vi "Launch Storage Line.vi"(8 "error in (no error)":errorcluster, 11 "cRIO-CO2 in":refnum<class "cRIO-CO2.lvclass">) -> (0 "error out":errorcluster, 3 "cRIO-CO2 out":refnum<class "cRIO-CO2.lvclass">)   [LabVIEW 2015, in "cRIO-Carbondioxide.lvlib" / "cRIO-CO2.lvlib" / "cRIO-CO2.lvclass"]
uses:
  cRIO-CO2.lvclass
  Storage Line/Storage Line.lvclass
  CO2 Actor/CO2 Actor.lvclass
  <vilib>/ActorFramework/Actor/Actor.lvclass
  cRIO-CO2.lvclass/cRIO-CO2.ctl
  cRIO-CO2 Messages/Log Message Msg/Log Message Msg.lvclass/Log Message Msg.ctl
  <vilib>/ActorFramework/Message Enqueuer/Message Enqueuer.lvclass/Message Enqueuer.ctl
  <vilib>/ActorFramework/Message Enqueuer/Enqueue.vi
  <vilib>/ActorFramework/Message Priority Queue/Priority Enqueue.vi
  <vilib>/ActorFramework/Message Enqueuer/Message Enqueuer.lvclass
  cRIO-CO2 Messages/Log Message Msg/Log Message Msg.lvclass
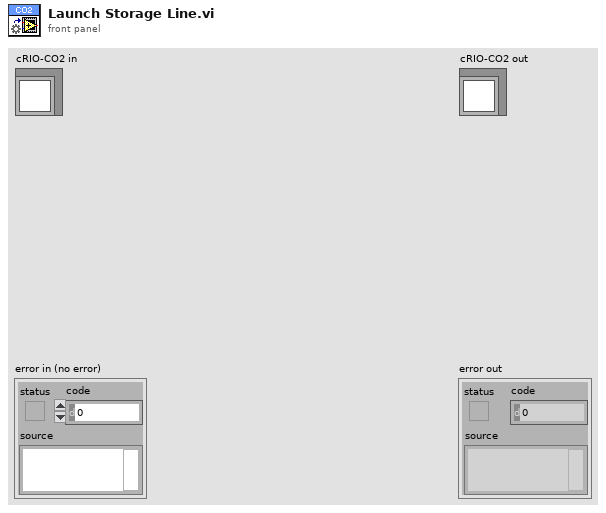
[diagram p1: front panel]
types:
  T1 = typedef "Dedicated Enqueuers.ctl" = cluster{"Freezers":cluster{"Syringe":refnum<class "Message Enqueuer.lvclass">, "Tank 1":refnum<class "Message Enqueuer.lvclass">, "Tank 2":refnum<class "Message Enqueuer.lvclass">, "Tank 3":refnum<class "Message Enqueuer.lvclass">, "Tank 4":refnum<class "Message Enqueuer.lvclass">}, "Heaters":cluster{"Syringe":refnum<class "Message Enqueuer.lvclass">, "Piston":refnum<class "Message Enqueuer.lvclass">}, "Blowers":cluster{"Tank 1":refnum<class "Message Enqueuer.lvclass">, "Tank 2":refnum<class "Message Enqueuer.lvclass">, "Tank 3":refnum<class "Message Enqueuer.lvclass">, "Tank 4":refnum<class "Message Enqueuer.lvclass">, "Syringe":refnum<class "Message Enqueuer.lvclass">}, "Sample Line":refnum<class "Message Enqueuer.lvclass">, "Storage Line":refnum<class "Message Enqueuer.lvclass">, "Transfer Line":refnum<class "Message Enqueuer.lvclass">, "Syringe Stepper":refnum<class "Message Enqueuer.lvclass">, "Syringe Line":refnum<class "Message Enqueuer.lvclass">, "Capillary Line":refnum<class "Message Enqueuer.lvclass">, "Preparation Line":refnum<class "Message Enqueuer.lvclass">, "Turbo":refnum<class "Message Enqueuer.lvclass">, "Vacuum":refnum<class "Message Enqueuer.lvclass">, "He Line":refnum<class "Message Enqueuer.lvclass">, "Cylinder":refnum<class "Message Enqueuer.lvclass">}
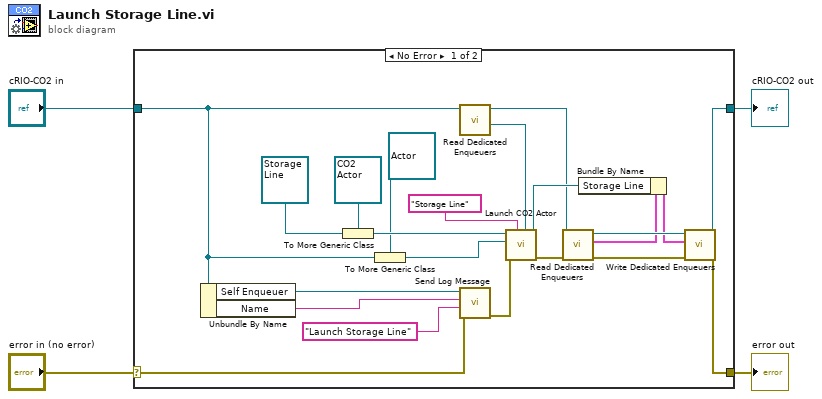
[diagram p0: block diagram]
diagram:
  n1 = case shown="No Error" "error in (no error)" {
    selector: "error in (no error)" -> [w23 w28]
    tunnel: [w11 w28] -> w3
    tunnel: [w13 w27] -> w1
    tunnel: "cRIO-CO2 in" -> [w9 w27]
    frame No Error {
      n2 = Unbundle By Name(w9) -> ("Self Enqueuer"=w10:refnum<class "Message Enqueuer.lvclass">, "Name"=w20:string)
      n3 = To More Generic Class(target class=refnum<class "CO2 Actor.lvclass"> refnum ("CO2 Actor in"), reference=refnum<class "Storage Line.lvclass"> refnum ("Storage Line.lvclass")) -> (generic class reference=w25:refnum<class "CO2 Actor.lvclass">)
      n4 = To More Generic Class(target class=refnum<class "Actor.lvclass"> refnum ("Caller Actor in"), reference=w9) -> (generic class reference=w7:refnum<class "Actor.lvclass">)
      n5 = call "Read Dedicated Enqueuers.vi"("cRIO-CO2 in"=w9) -> ("Qs.DedicatedEnQrs"=w5:refnum<queue>, "cRIO-CO2 out"=w6:refnum<class "cRIO-CO2.lvclass">)  [unwired: 7 in, 2 out]
      n6 = call "Send Log Message.vi"("error in (no error)"=w23, "String"="Launch Storage Line", "Source Name"=w20, "Message Enqueuer"=w10) -> ("error out"=w22:errorcluster)  [unwired: 6 in, 1 out]
      n7 = call "Launch CO2 Actor.vi"("DedicatedEnQrs"=w5, "Name"="Storage Line", "error in (no error)"=w22, "Caller Actor in"=w7, "CO2 Actor in"=w25) -> ("error out"=w12:errorcluster, "Caller-To-Actor Enqueuer"=w18:refnum<class "Message Enqueuer.lvclass">)  [unwired: 5 in]
      n8 = call "Read Dedicated Enqueuers.vi"("error in (no error)"=w12, "cRIO-CO2 in"=w6) -> ("error out"=w17:errorcluster, "Dedicated Enqueuers"=w15:T1, "cRIO-CO2 out"=w16:refnum<class "cRIO-CO2.lvclass">)  [unwired: 6 in, 1 out]
      n9 = Bundle By Name(cluster=w15, "Storage Line"=w18) -> (w14:T1)
      n10 = call "Write Dedicated Enqueuers.vi"("error in (no error)"=w17, "Dedicated Enqueuers"=w14, "cRIO-CO2 in"=w16) -> ("error out"=w11:errorcluster, "cRIO-CO2 out"=w13:refnum<class "cRIO-CO2.lvclass">)  [unwired: 7 in]
    }
    frame Error {
    }
  }
  "error out" <- w3
  "cRIO-CO2 out" <- w1
